vi "Error Engine - Strip Path.vi"(7 "Strip Lib App Types":T1(ring), 8 "error in (no error)":errorcluster, 11 "File Path In":path) -> (0 "error out":errorcluster, 3 "Stripped File Path":path)   [LabVIEW 2023, in "Error_Engine_Actor.lvlib" / "Error_Emgime_Class.lvclass"]
uses:
  Error_Emgime_Class.lvclass
  <vilib>/Utility/error.llb/Trim Whitespace One-Sided.vi
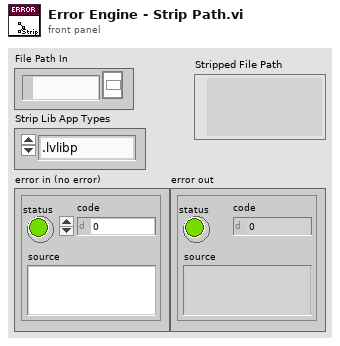
[diagram p1: front panel]
types:
  T1 = enum16{".lvlibp", ".exe", ".llb", "Calling all from .exe"}
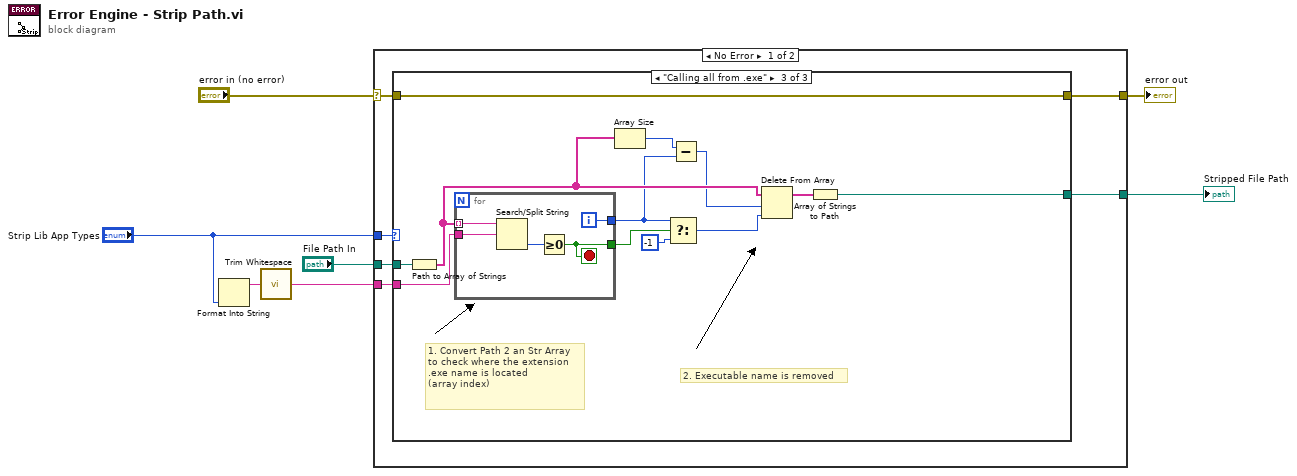
[diagram p0: block diagram]
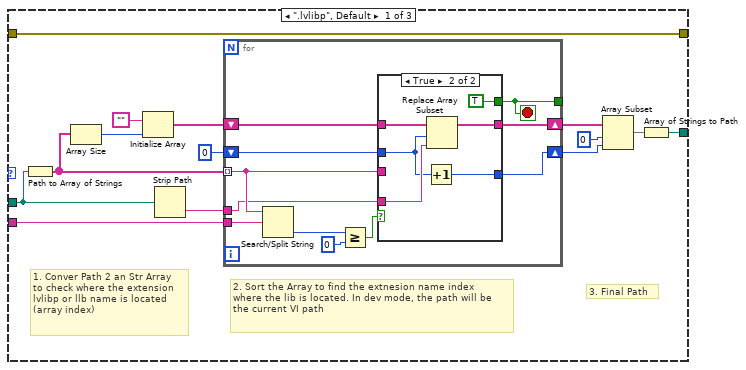
[diagram p2: hidden frame]
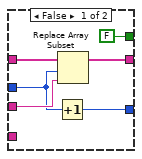
[diagram p3: hidden frame]
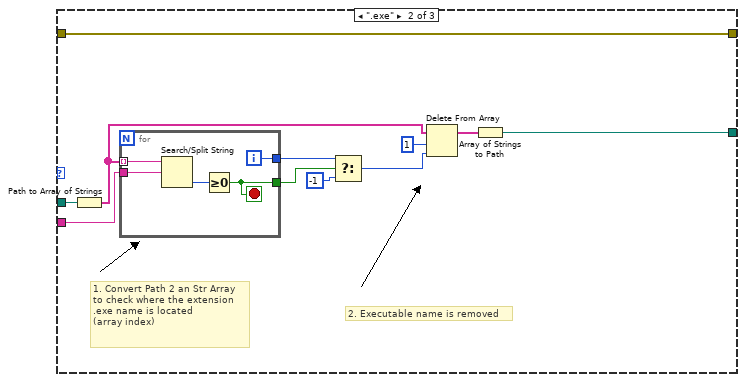
[diagram p4: hidden frame]
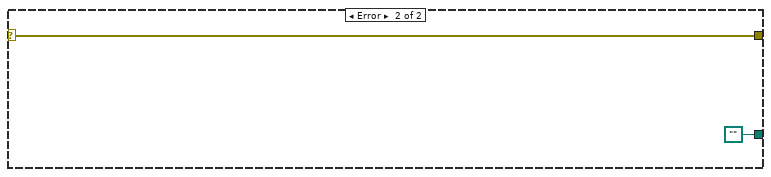
[diagram p5: hidden frame]
diagram:
  n1 = Format Into String("Strip Lib App Types") -> (resulting string=w3:string)  [unwired: 3 in, 1 out]
  n2 = call <vilib>:"Trim Whitespace.vi"("string"=w3) -> ("trimmed string"=w1:string)  [unwired: 1 in]
  n3 = case shown="No Error" "error in (no error)" {
    selector: "error in (no error)" -> [w9 w85]
    tunnel: "File Path In" -> [w13 _]
    tunnel: [w11 path "" ("path")] -> w5
    tunnel: [w8 w85] -> w6
    tunnel: w1 -> [w12 _]
    tunnel: "Strip Lib App Types" -> [w10 _]
    frame No Error {
      n4 = case shown="\"Calling all from .exe\"" w10 {
        tunnel: w13 -> [w17 w61 w78]
        tunnel: w12 -> [w16 w60 w77]
        tunnel: [w14 w57 w75] -> w11
        tunnel: w9 -> [w15 w51 w71]
        tunnel: [w15 w51 w71] -> w8
        frame ".lvlibp", Default {
          # "3. Final Path"
          # "2. Sort the Array to find the extnesion name index\nwhere the lib is located. In dev mode, the path will be\nthe current VI path"
          # "1. Conver Path 2 an Str Array\nto check where the extension\nlvlibp or llb name is located \n(array index)"
          n5 = Path to Array of Strings(0:w17) -> (2:w25:string[])  [unwired: 1 out]
          n6 = Array Size(array=w25) -> (size(s)=w24:i32)
          n7 = Initialize Array("", w24) -> (w26:string[])
          n8 = Strip Path(path=w17) -> (name=w22:string)  [unwired: 1 out]
          n9 = for {
            tunnel: w25 -> [w34] mode=indexing
            shift-right: [w33] -> w18
            shift-left: w26 -> [w35]
            shift-right: [w31] -> w19
            shift-left: 0 -> [w32]
            tunnel: [w30] -> _
            tunnel: w22 -> [w29]
            tunnel: w16 -> [w28]
            stop <- w30 stop-if-true
            n10 = Search/Split String(string=w34, search string/char (-)=w28) -> (offset of match=w38:i32)  [unwired: 1 in, 2 out]
            n11 = Greater Or Equal?(x=w38, y=0) -> (x >= y?=w36:bool)
            n12 = case shown="True" w36 {
              tunnel: w35 -> [w44 w49]
              tunnel: w34 -> [w43 _]
              tunnel: [w40 w45] -> w33
              tunnel: w32 -> [w41 w47]
              tunnel: [w42 w46] -> w31
              tunnel: [FALSE TRUE] -> w30
              tunnel: w29 -> [_ w48]
              frame False {
                n13 = Increment(x=w41) -> (x+1=w42:i32)
                n14 = Replace Array Subset(array=w44, new element=w43, index=w41) -> (w40:string[])
              }
              frame True {
                n15 = Increment(x=w47) -> (x+1=w46:i32)
                n16 = Replace Array Subset(array=w49, new element=w48, index=w47) -> (w45:string[])
              }
            }
          }
          n17 = Array Subset(array=w18, index=0, length=w19) -> (w20:string[])
          n18 = Array of Strings to Path(0:w20) -> (2:w14:path)  [unwired: 1 in]
        }
        frame ".exe" {
          # "2. Executable name is removed"
          # "1. Convert Path 2 an Str Array\nto check where the extension\n.exe name is located \n(array index)"
          n19 = Path to Array of Strings(0:w61) -> (2:w58:string[])  [unwired: 1 out]
          n20 = for {
            tunnel: w58 -> [w66] mode=indexing
            tunnel: w60 -> [w65]
            tunnel: [w64] -> w54
            tunnel: [w62] -> w55
            i -> [w64]
            stop <- w62 stop-if-true
            n21 = Search/Split String(string=w66, search string/char (-)=w65) -> (offset of match=w63:i32)  [unwired: 1 in, 2 out]
            n22 = Greater Or Equal To 0?(x=w63) -> (x >= 0?=w62:bool)
          }
          n23 = Select(t=w54, s=w55, f=-1 ("index")) -> (s? t:f=w52:i32)
          n24 = Delete From Array(array=w58, length=1, index=w52) -> (array with subset deleted=w59:string[])  [unwired: 1 out]
          n25 = Array of Strings to Path(0:w59) -> (2:w57:path)  [unwired: 1 in]
        }
        frame "Calling all from .exe" {
          # "2. Executable name is removed"
          # "1. Convert Path 2 an Str Array\nto check where the extension\n.exe name is located \n(array index)"
          n26 = Path to Array of Strings(0:w78) -> (2:w70:string[])  [unwired: 1 out]
          n27 = for {
            tunnel: w70 -> [w83] mode=indexing
            tunnel: w77 -> [w82]
            tunnel: [w81] -> w68
            tunnel: [w79] -> w74
            i -> [w81]
            stop <- w79 stop-if-true
            n28 = Search/Split String(string=w83, search string/char (-)=w82) -> (offset of match=w80:i32)  [unwired: 1 in, 2 out]
            n29 = Greater Or Equal To 0?(x=w80) -> (x >= 0?=w79:bool)
          }
          n30 = Array Size(array=w70) -> (size(s)=w69:i32)
          n31 = Select(t=w68, s=w74, f=-1 ("index")) -> (s? t:f=w72:i32)
          n32 = Subtract(x=w69, y=w68) -> (x-y=w67:i32)
          n33 = Delete From Array(array=w70, length=w67, index=w72) -> (array with subset deleted=w76:string[])  [unwired: 1 out]
          n34 = Array of Strings to Path(0:w76) -> (2:w75:path)  [unwired: 1 in]
        }
      }
    }
    frame Error {
    }
  }
  "Stripped File Path" <- w5
  "error out" <- w6
